vi "ClearAllTree.vi"(8 "error in (no error)":errorcluster, 11 "ClassDataTree in":refnum<class "ClassDataTree.lvclass">) -> (0 "error out":errorcluster, 3 "ClassDataTree out":refnum<class "ClassDataTree.lvclass">)   [LabVIEW 2010, in "ClassDataTree.lvclass"]
uses:
  ClassDataTree.lvclass
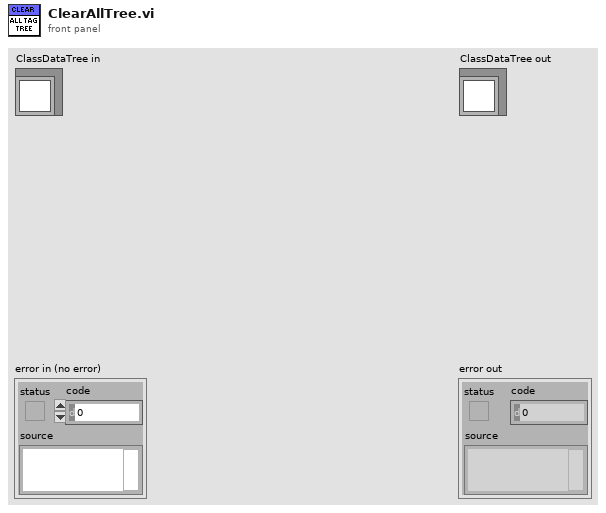
[diagram p1: front panel]
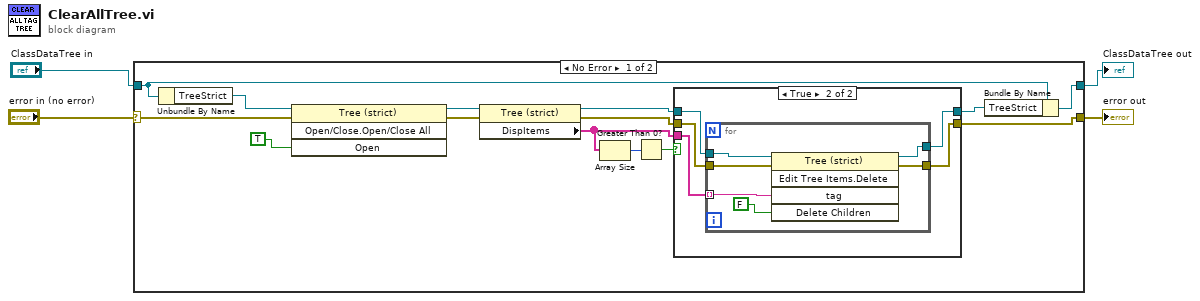
[diagram p0: block diagram]
diagram:
  n1 = case shown="No Error" "error in (no error)" {
    selector: "error in (no error)" -> [w10 w33]
    tunnel: [w16 w33] -> w3
    tunnel: [w13 w32] -> w1
    tunnel: "ClassDataTree in" -> [w15 w32]
    frame No Error {
      n2 = Unbundle By Name(w15) -> ("TreeStrict"=w11:refnum<vi>)
      n3 = invoke class="Tree (strict)" method="Open/Close.Open/Close All"(reference=w11, error in=w10, "Open"=TRUE ("Open?")) -> (reference out=w9:refnum<vi>, error out=w8:errorcluster)  [unwired: 1 in, 2 out]
      n4 = property class="Tree (strict)"(reference=w9, error in=w8) -> (reference out=w18:refnum<vi>, error out=w17:errorcluster, "DispItems"=w7:string[])
      n5 = Array Size(array=w7) -> (size(s)=w6:i32)
      n6 = Greater Than 0?(x=w6) -> (x > 0?=w5:bool)
      n7 = case shown="True" w5 {
        tunnel: w18 -> [w20 w25]
        tunnel: w17 -> [w19 w24]
        tunnel: w7 -> [_ w23]
        tunnel: [w19 w22] -> w16
        tunnel: [w20 w21] -> w14
        frame False {
        }
        frame True {
          n8 = for {
            tunnel: w25 -> [w31]
            tunnel: w24 -> [w30]
            tunnel: w23 -> [w28] mode=indexing
            tunnel: [w27] -> w21
            tunnel: [w26] -> w22
            n9 = invoke class="Tree (strict)" method="Edit Tree Items.Delete"(reference=w31, error in=w30, "tag"=w28, "Delete Children"=FALSE ("Delete Children?")) -> (reference out=w27:refnum<vi>, error out=w26:errorcluster)  [unwired: 1 in, 3 out]
          }
        }
      }
      n10 = Bundle By Name(cluster=w15, "TreeStrict"=w14) -> (w13:refnum<class "ClassDataTree.lvclass">)
    }
    frame Error {
    }
  }
  "error out" <- w3
  "ClassDataTree out" <- w1
